vi "Telescope Stop.vi"(8 "error in (no error)":errorcluster, 11 "LDT Telescope in":refnum<class "LDT Telescope.lvclass">) -> (0 "error out":errorcluster, 3 "LDT Telescope out":refnum<class "LDT Telescope.lvclass">)   [LabVIEW 2022 SP3, in "LDT Telescope.lvclass"]
uses:
  LDT Telescope.lvclass
  Telescope.lvclass
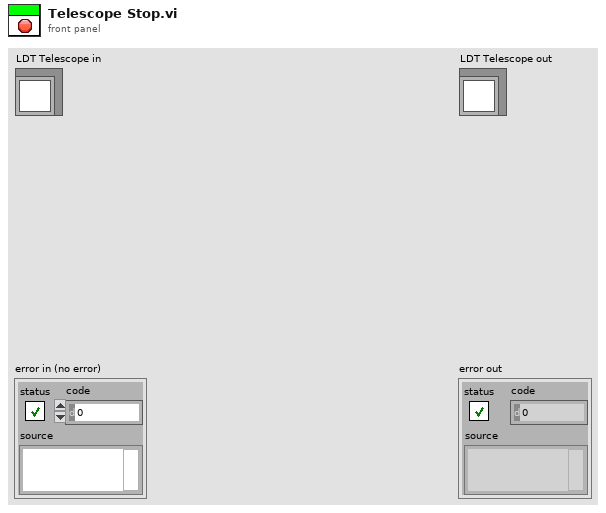
[diagram p1: front panel]
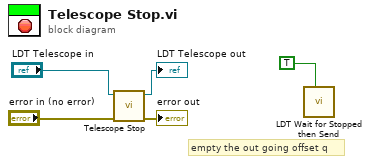
[diagram p0: block diagram]
diagram:
  # "empty the out going offset q"
  n1 = call-parent "Telescope Stop.vi"("error in (no error)"="error in (no error)", "Telescope in"="LDT Telescope in") -> ("error out"=→"error out":errorcluster, "Telescope out"=→"LDT Telescope out":refnum<class "LDT Telescope.lvclass">)  [unwired: 8 in]
  n2 = call "LDT Wait for Stopped then Send.vi"("add to q"=TRUE) -> ()  [unwired: 10 in, 1 out]
